vi "Get Available Font Encoding [ ].vi"(5 "Font path":path=path "C:/Windows/Fonts/ARIALUNI.TTF", 7 "Encoding":string="Identity-H", 11 "error in (no error)":errorcluster) -> (6 "CodePagesSupported [ ]":string[](array[string])=["1252 Latin 1", "1250 Latin 2: Eastern Europe", "1251 Cyrillic", "1253 Greek", "1254 Turkish", "1255 Hebrew", "1256 Arabic", "1257 Windows Baltic", "1258 Vietnamese", "874 Thai", "932 JIS/Japan", "936 Chinese: Simplified chars--PRC and Singapore", "949 Korean Wansung", "950 Chinese: Traditional chars--Taiwan and Hong Kong", "1361 Korean Johab", "Macintosh Character Set (US Roman)", "OEM Character Set", "869 IBM Greek", "866 MS-DOS Russian", "865 MS-DOS Nordic", "864 Arabic", "863 MS-DOS Canadian French", "862 Hebrew", "861 MS-DOS Icelandic", "860 MS-DOS Portuguese", "857 IBM Turkish", "855 IBM Cyrillic; primarily Russian", "852 Latin 2", "775 MS-DOS Baltic", "737 Greek; former 437 G", "708 Arabic; ASMO 708", "850 WE/Latin 1", "437 US"], 8 "Number CodePagesSupported":i32=33, 15 "error out":errorcluster)   [LabVIEW 2020, in "Exaprom PDF.lvlib"]
doc: "Version 1.1\nDeveloped by Jean-Marc Simard\nCopyright © 2012, Exaprom Inc.\nAll rights reserved.\nLicense: BSD\n\nWith iTextSharp 4.1.6 (http://itextsharp.sourceforge.net)\nunder Mozilla Public License Version 1.1\n(http://www.mozilla.org/MPL/MPL-1.1.html)"
uses:
  <userlib>/labview-PDF-writer-master/Exaprom PDF.lvlib
  C:/Program Files (x86)/National Instruments/LabVIEW 2020/user.lib/labview-PDF-writer-master/DLL/itextsharp.dll
  DLL/itextsharp.dll
panel:
  out "元素":refnum<k24>
  # "You nedd to know, at least, one encoding!"
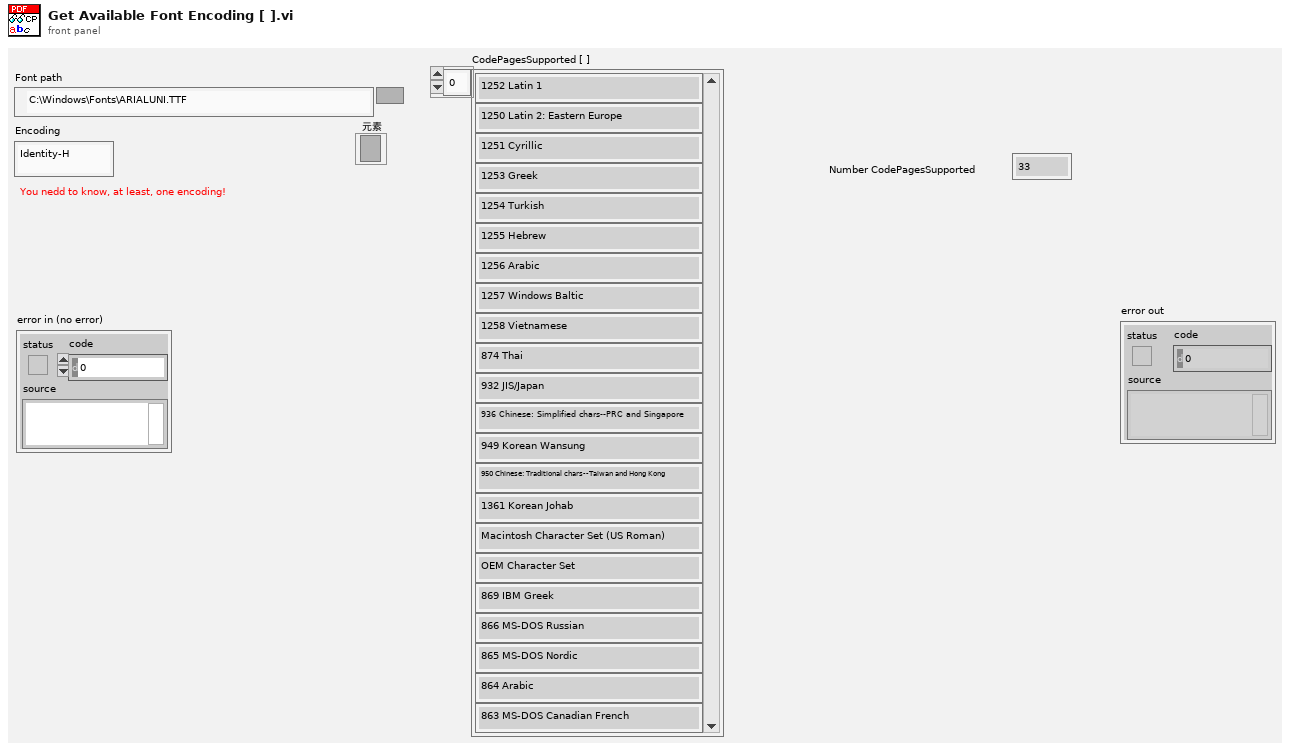
[diagram p1: front panel]
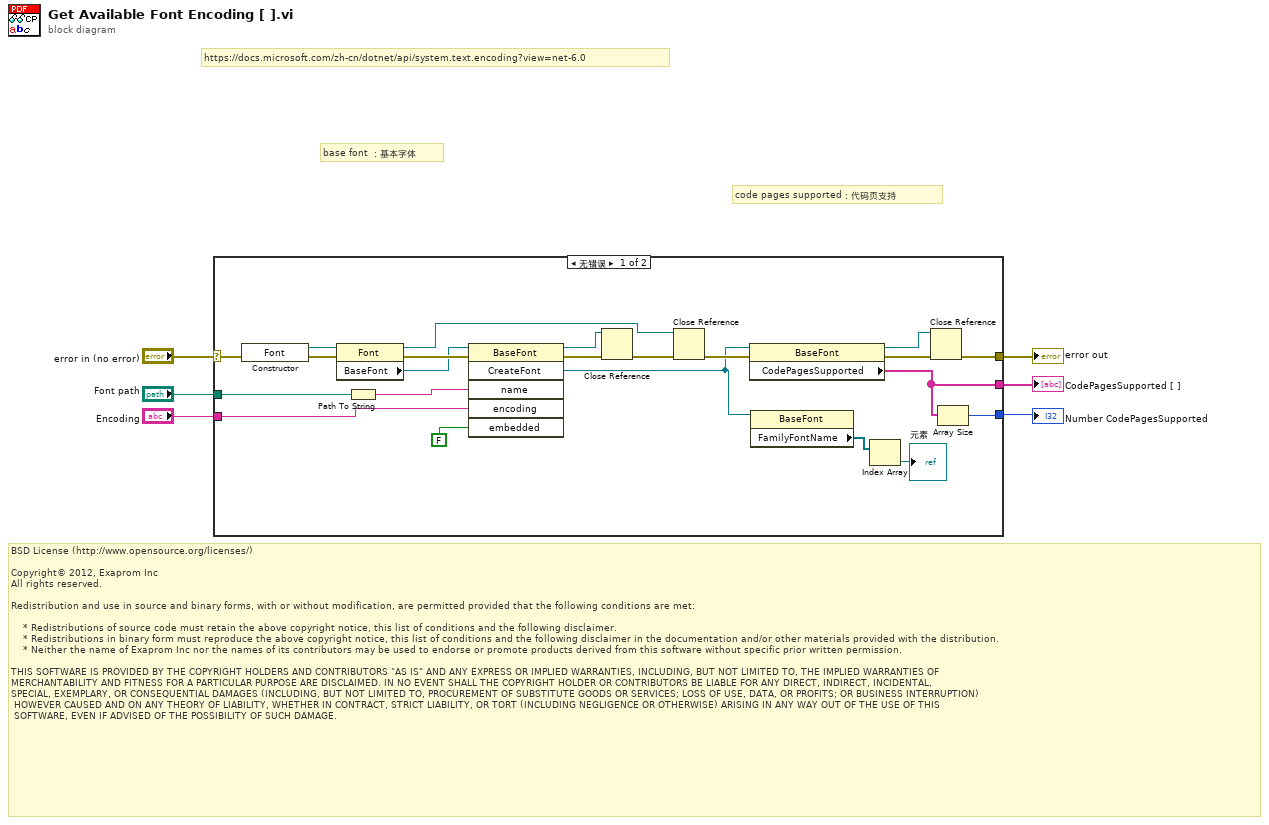
[diagram p0: block diagram]
diagram:
  # "https://docs.microsoft.com/zh-cn/dotnet/api/system.text.encoding?view=net-6.0"
  # "code pages supported：代码页支持"
  # "base font ：基本字体"
  # "BSD License (http://www.opensource.org/licenses/)\n\nCopyright© 2012, Exaprom Inc\nAll rights reserved.\n\nRedistribution and use in source and binary forms, with or without modification, are permitted provided that the following conditions are met:\n\n    * Redistributions of source code must retain the above copyright notice, this list of conditions and the following disclaimer.\n    * Redistributions in binary form must reproduce the above copyright notice, this list of conditions and the following disclaimer in the documentation and/or other materials provided with the distribution.\n    * Neither the name of Exaprom Inc nor the names of its contributors may be used to endorse or promote products derived from this software without specific prior written permission.\n\nTHIS SOFTWARE IS PROVIDED BY THE COPYRIGHT HOLDERS AND CONTRIBUTORS \"AS IS\" AND ANY EXPRESS OR IMPLIED WARRANTIES, INCLUDING, BUT NOT LIMITED TO, THE IMPLIED WARRANTIES OF \nMERCHANTABILITY AND FITNESS FOR A PARTICULAR PURPOSE ARE DISCLAIMED. IN NO EVENT SHALL THE COPYRIGHT HOLDER OR CONTRIBUTORS BE LIABLE FOR ANY DIRECT, INDIRECT, INCIDENTAL,\nSPECIAL, EXEMPLARY, OR CONSEQUENTIAL DAMAGES (INCLUDING, BUT NOT LIMITED TO, PROCUREMENT OF SUBSTITUTE GOODS OR SERVICES; LOSS OF USE, DATA, OR PROFITS; OR BUSINESS INTERRUPTION)\n HOWEVER CAUSED AND ON ANY THEORY OF LIABILITY, WHETHER IN CONTRACT, STRICT LIABILITY, OR TORT (INCLUDING NEGLIGENCE OR OTHERWISE) ARISING IN ANY WAY OUT OF THE USE OF THIS\n SOFTWARE, EVEN IF ADVISED OF THE POSSIBILITY OF SUCH DAMAGE."
  n1 = case shown="无错误" "error in (no error)" {
    selector: "error in (no error)" -> [w24 w29]
    tunnel: [w13 w29] -> w6
    tunnel: "Font path" -> [w23 _]
    tunnel: "Encoding" -> [w21 _]
    tunnel: [w15 _] -> w2
    tunnel: [w16 _] -> w1
    frame No Error {
      n2 = constructor class="Font"(error in=w24) -> (reference out=w28:refnum<k24>, error out=w27:errorcluster)  [unwired: 2 in, 1 out]
      n3 = property class="Font"(reference=w28, error in=w27) -> (reference out=w18:refnum<k24>, error out=w26:errorcluster, "BaseFont"=w11:refnum<k24>)
      n4 = Path To String(path=w23) -> (string=w22:string)
      n5 = invoke class="BaseFont" method="CreateFont"(reference=w11, error in=w26, "name"=w22, "encoding"=w21, "embedded"=FALSE) -> (reference out=w10:refnum<k24>, error out=w25:errorcluster, "CreateFont"=w9:refnum<k24>)  [unwired: 1 in, 3 out]
      n6 = Close Reference(reference=w10, error in (no error)=w25) -> (error out=w19:errorcluster)
      n7 = Close Reference(reference=w18, error in (no error)=w19) -> (error out=w17:errorcluster)
      n8 = property class="BaseFont"(reference=w9, error in=w17) -> (reference out=w12:refnum<k24>, error out=w14:errorcluster, "CodePagesSupported"=w15:string[])
      n9 = property class="BaseFont"(reference=w9) -> ("FamilyFontName"=w8:refnum<k24>[])  [unwired: 1 in, 2 out]
      n10 = Index Array(array=w8) -> (element=→"元素":refnum<k24>)  [unwired: 1 in]
      n11 = Close Reference(reference=w12, error in (no error)=w14) -> (error out=w13:errorcluster)
      n12 = Array Size(array=w15) -> (size(s)=w16:i32)
    }
    frame Error {
    }
  }
  "error out" <- w6
  "CodePagesSupported [ ]" <- w2
  "Number CodePagesSupported" <- w1
